vi "labview1.vi"() -> ()   [LabVIEW 2022 SP3]
panel:
  out "Waveform Graph":dbl[](graph)
  out "Array":dbl[](array[numeric])
  in  "Noise":dbl
  in  "offset":dbl
  in  "Amplitude":dbl
  in  "Nb de points":i32
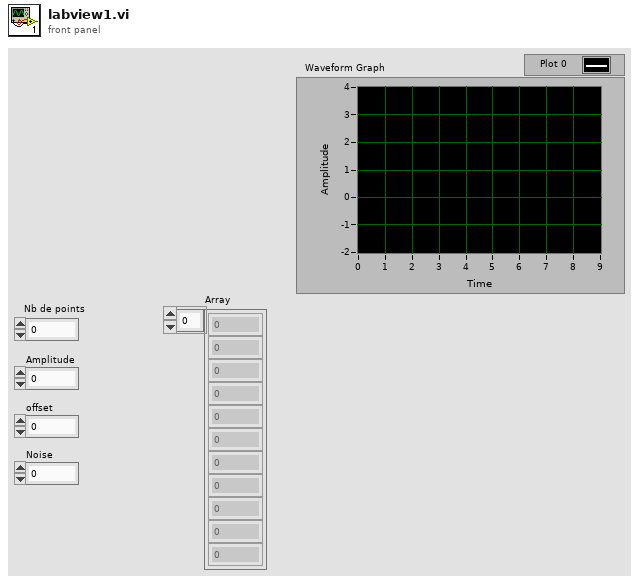
[diagram p1: front panel]
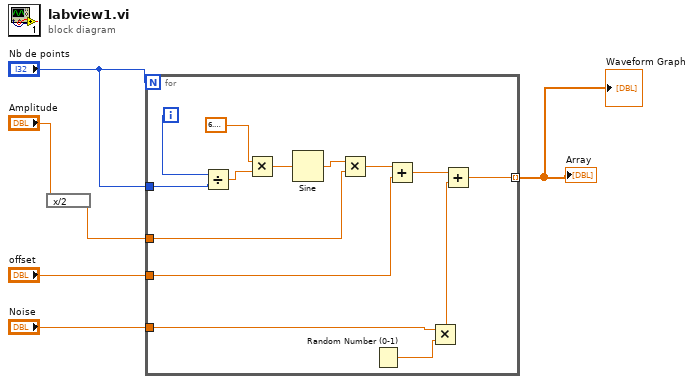
[diagram p0: block diagram]
diagram:
  n1 = expression code="x/2"("Amplitude") -> (w4:dbl)
  n2 = for {
    N: "Nb de points" -> [_]
    tunnel: "Nb de points" -> [w19]
    tunnel: w4 -> [w13]
    tunnel: [w11] -> w1 mode=indexing
    tunnel: "offset" -> [w10]
    tunnel: "Noise" -> [w9]
    i -> [w20]
    n3 = Divide(x=w20, y=w19) -> (x/y=w18:dbl)
    n4 = Multiply(x=6.283185307179586, y=w18) -> (x*y=w17:dbl)
    n5 = Sine(x=w17) -> (sin(x)=w16:dbl)
    n6 = Multiply(x=w16, y=w13) -> (x*y=w15:dbl)
    n7 = Random Number (0-1)() -> (number: 0 to 1=w7:dbl)
    n8 = Add(x=w15, y=w10) -> (x+y=w12:dbl)
    n9 = Multiply(x=w9, y=w7) -> (x*y=w8:dbl)
    n10 = Add(x=w12, y=w8) -> (x+y=w11:dbl)
  }
  "Array" <- w1
  "Waveform Graph" <- w1
